vi "Add Shared Variables.vi"(8 "error in (no error)":errorcluster, 11 "Node Ptr":u64 format="%.0x") -> (0 "error out":errorcluster)   [LabVIEW 2017]
uses:
  Support/Add SV Process/Channel Configuration States.ctl
  Support/ChannelVS/ChannelVS.lvclass
  C:/Users/Public/Documents/National Instruments/NI VeriStand 2017/Custom Devices/Shared Variables CD 2.0/Data/Channel.lvlibp/Channel.lvclass
  <vilib>/Utility/VariantDataType/Type.ctl
  Support/ChannelVS/ChannelVS.lvclass/ChannelVS.ctl
  Support/ChannelVS/Compare Ch with Ch List.vi
  Support/ChannelVS/Read VeriSTAND Channel Info.vi
  Support/ChannelVS/Write VeriSTAND Channel Info.vi
  Shared/SV Global.vi
  Public/Documents/National Instruments/NI VeriStand 2017/Custom Devices/Shared Variables CD 2.0/Data/Channel.lvlibp/Read Channel Info.vi
  <vilib>/NI VeriStand/Custom Device API/Custom Device API.lvlib
  Shared Variables CD 2.0 Configuration.lvlib
  <vilib>/Utility/VariantDataType/VariantType.lvlib
panel:
  out "Scope":string
  out "State":T1
  in  "Refresh Target":bool
  in  "Done":bool
  in  "Help":bool
  in  "Remove Button":bool
  in  "Add Button":bool
  in  "Target IPAddr":string caption="Target IP Address*"
  in  "CD List":string[](tree)
  in  "Target List":string[](tree)
  in  "Tag":string
  # "Manage Shared Variables to"
  # "*Do Not Use \"localhost\" or host name"
  # "*Grayed out variables are already added to Veristand"
  # "All Numeric data types will be handled as\nDouble Floating Point in VeriSTAND"
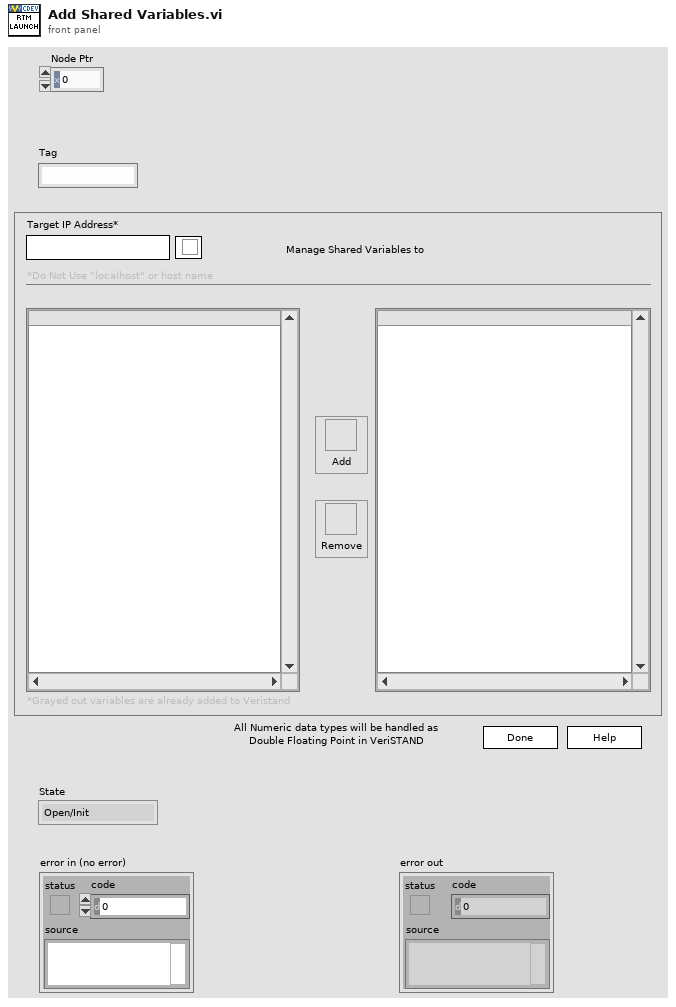
[diagram p1: front panel]
types:
  T1 = typedef "Shared Variables CD 2.0 Configuration.lvlib/Channel Configuration States.ctl" = enum16{"Open/Init", "Start Update", "Get VS Channels", "Get Available Ch from Target", "Wait On User Action", "Update Target Tree", "Update VS Trees", "Update Done", "Create VS Channels", "Remove VS Channels", "Error", "Close"}
  T2 = cluster{"Read Channel Array":refnum<class "ChannelVS.lvclass">[], "Write Channel Array":refnum<class "ChannelVS.lvclass">[]}
  T3 = typedef "Custom Device API.lvlib/Custom Device Item Info.ctl" = cluster{"Name":string, "Is Channel":bool, "GUID":string, "Is Waveform":bool}
  T4 = typedef "Custom Device API.lvlib/Custom Device Item Ref.ctl" = u64
  T5 = enum8{"Enabled", "Disabled", "Disabled and Grayed Out"}
  T6 = typedef "VariantType.lvlib/Type.ctl" = enum8{"Invalid Type", "Void", "I8", "I16", "I32", "I64", "U8", "U16", "U32", "U64", "Single Float", "Double Float", "Extended Float", "Single Complex", "Double Complex", "Extended Complex", "Enum U8", "Enum U16", "Enum U32", "Enum U64", "Single Float With Unit", "Double Float With Unit", "Extended Float With Unit", "Single Complex with Unit", "Double Complex with Unit", "Extended Complex with Unit", "Boolean", "String", "Path", "Picture", "Tag", "Array", "Cluster", "Variant", "LV Variant", "Waveform", "Timestamp", "Digital Waveform", "Digital Data", "ExpressData", "Refnum", "External Data", "VI", "Poly VI", "LabVIEW Class Instance", "Fixed Point"}
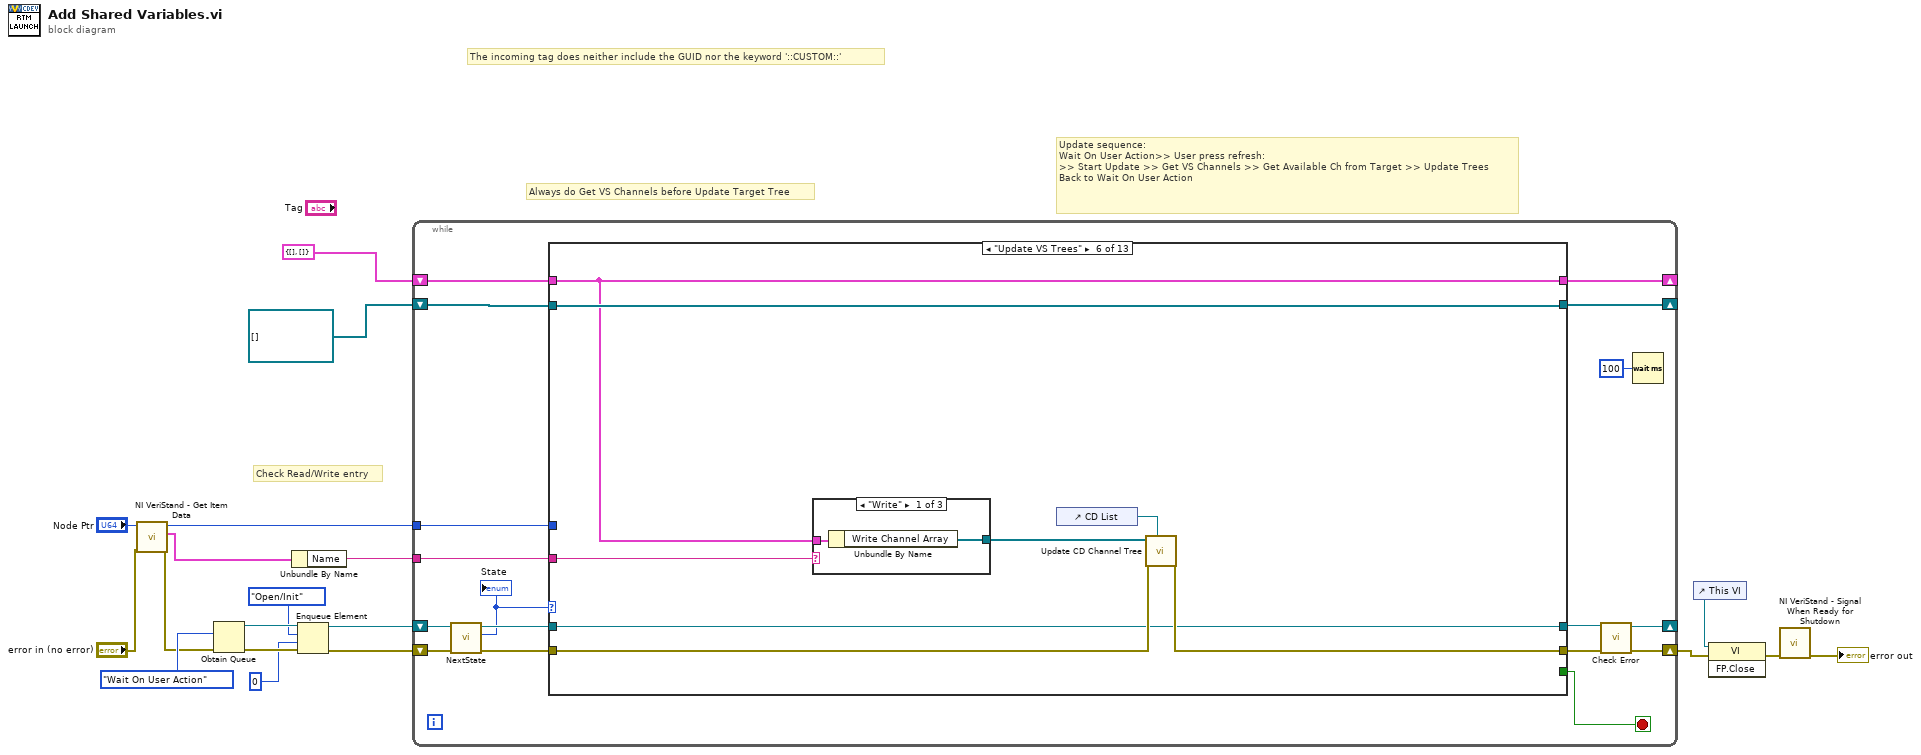
[diagram p0: block diagram]
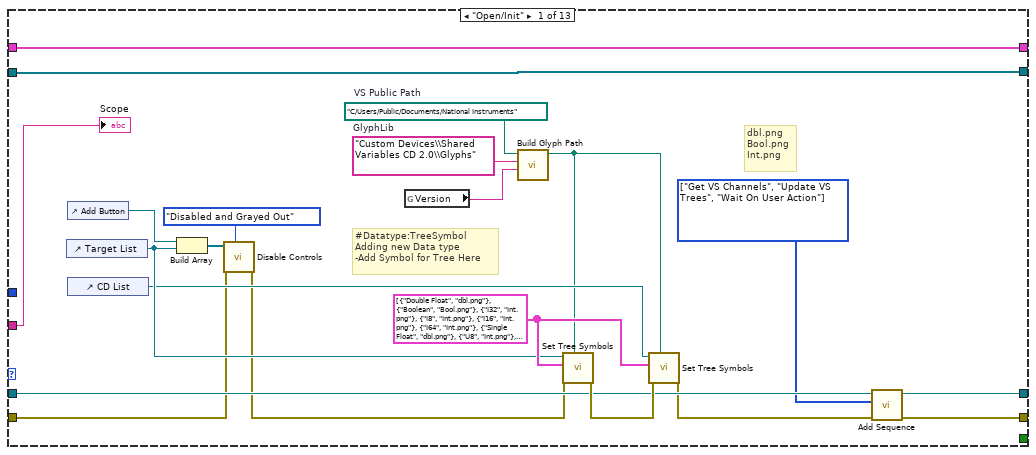
[diagram p2: hidden frame]
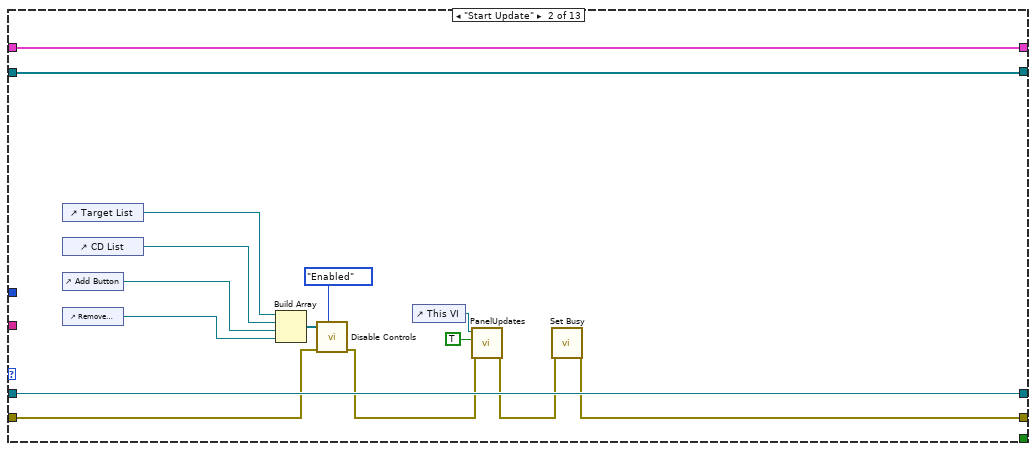
[diagram p3: hidden frame]
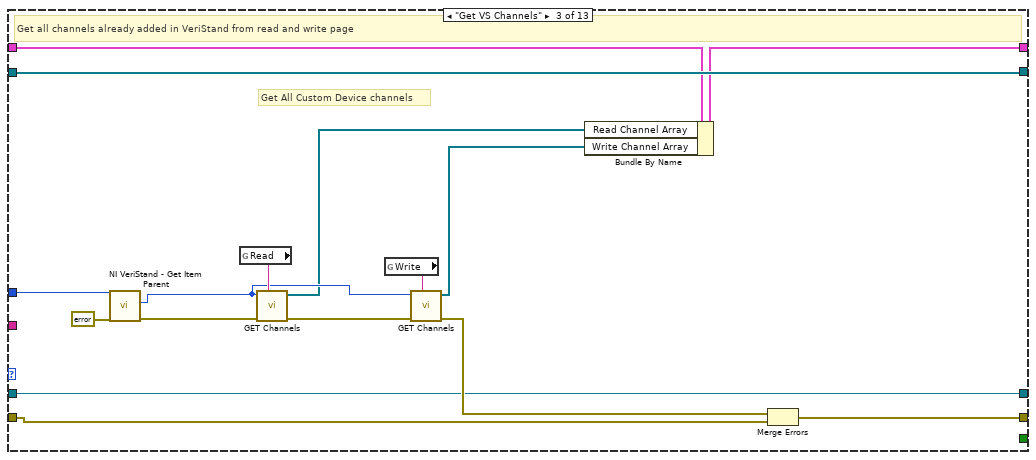
[diagram p4: hidden frame]
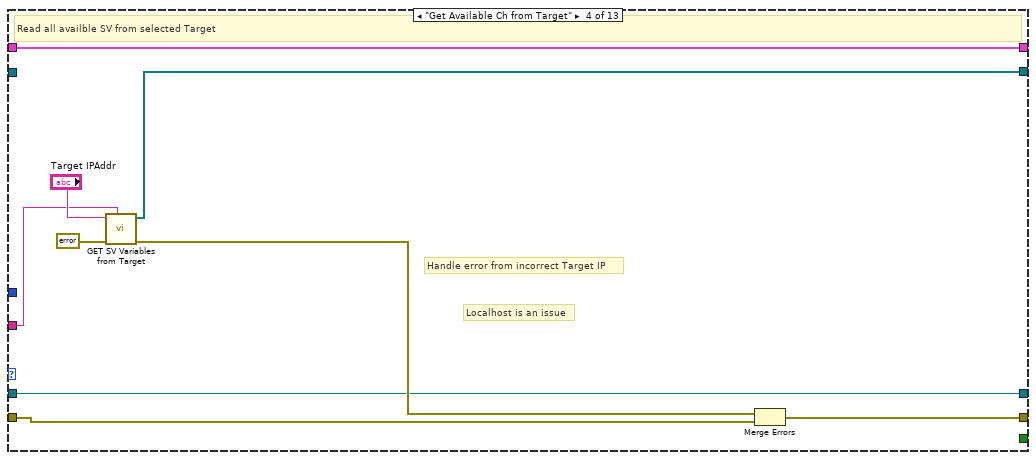
[diagram p5: hidden frame]
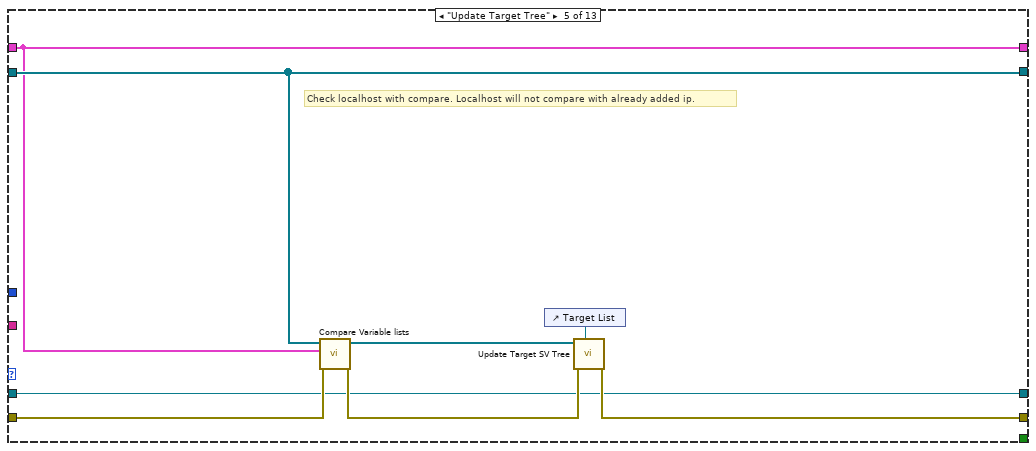
[diagram p6: hidden frame]
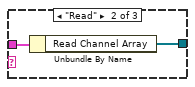
[diagram p7: hidden frame]
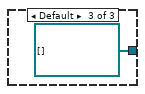
[diagram p8: hidden frame]
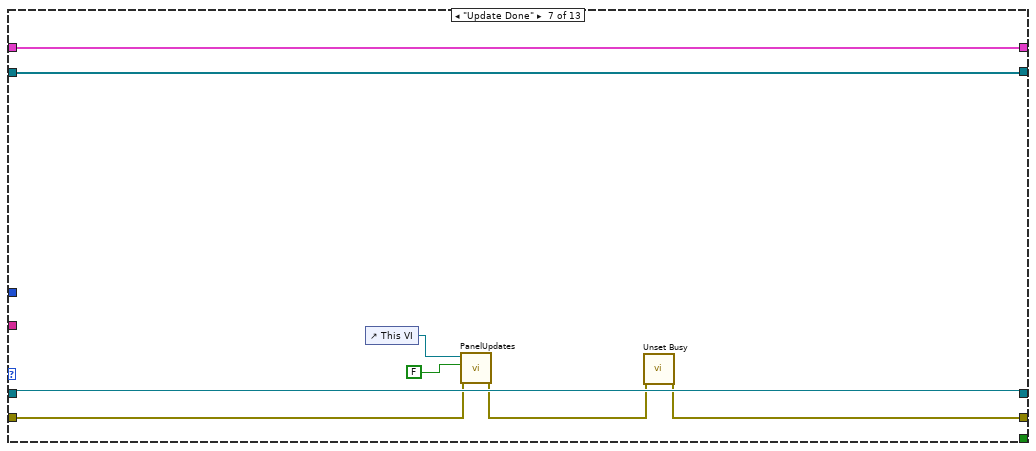
[diagram p9: hidden frame]
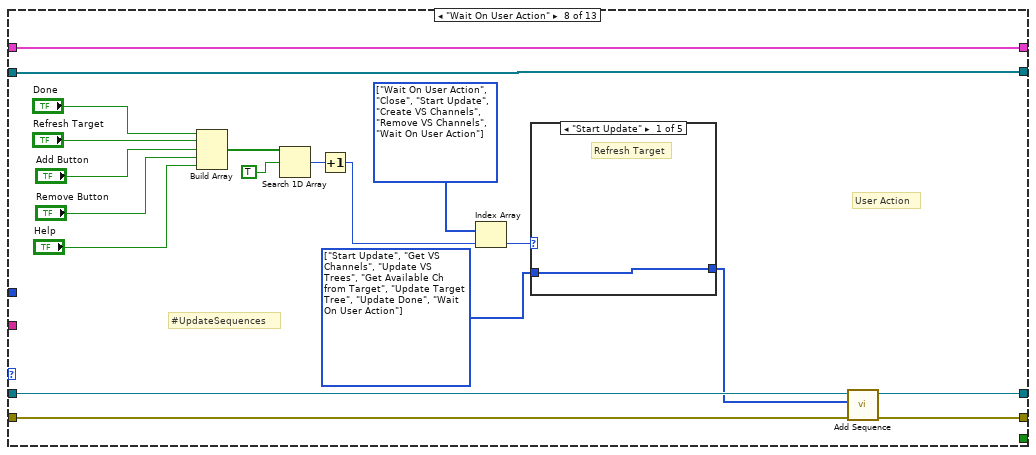
[diagram p10: hidden frame]
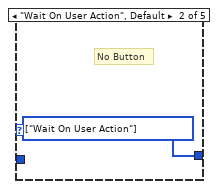
[diagram p11: hidden frame]
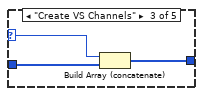
[diagram p12: hidden frame]
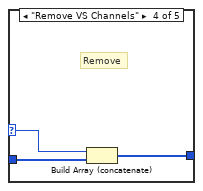
[diagram p13: hidden frame]
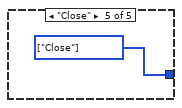
[diagram p14: hidden frame]
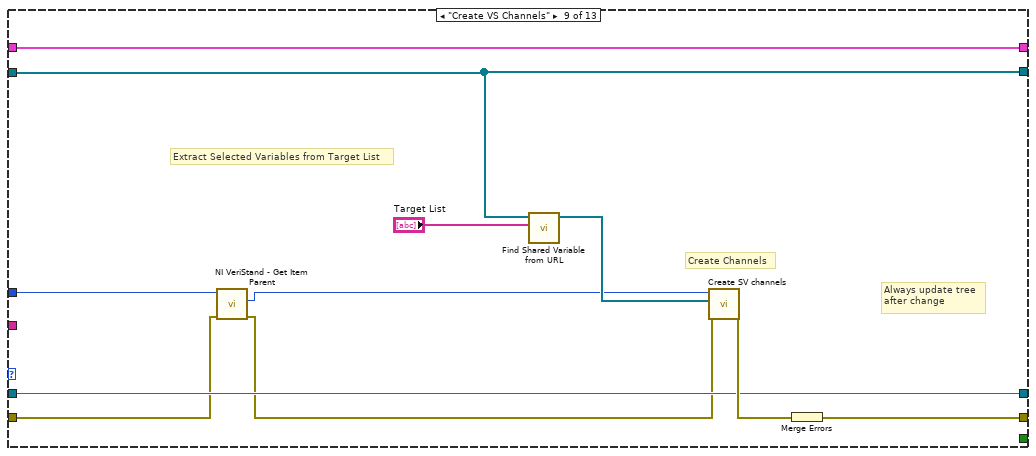
[diagram p15: hidden frame]
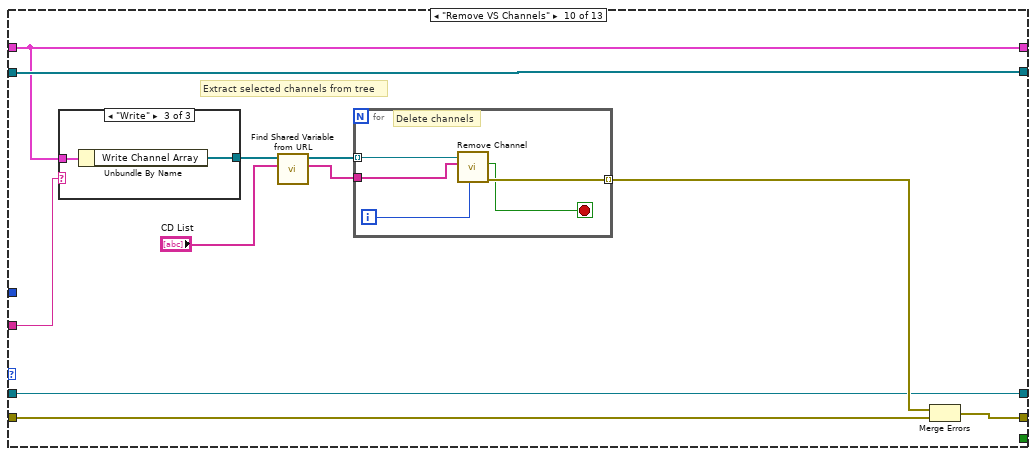
[diagram p16: hidden frame]
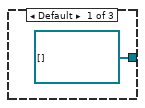
[diagram p17: hidden frame]
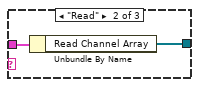
[diagram p18: hidden frame]
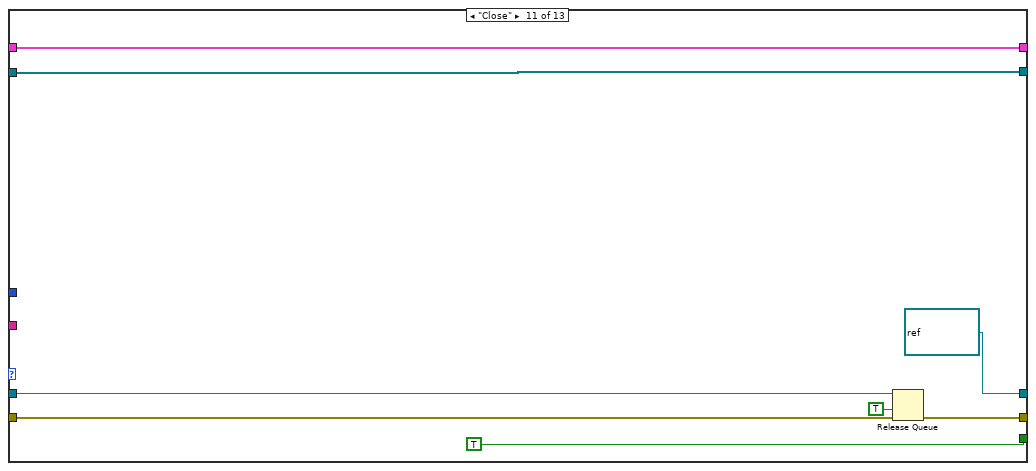
[diagram p19: hidden frame]
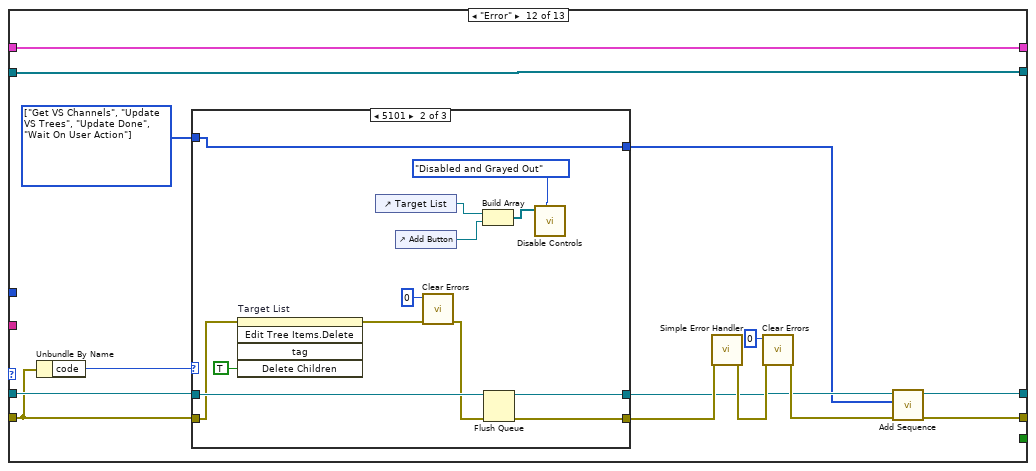
[diagram p20: hidden frame]
diagram:
  # "Always do Get VS Channels before Update Target Tree"
  # "Check Read/Write entry"
  # "Update sequence:\nWait On User Action>> User press refresh:\n>> Start Update >> Get VS Channels >> Get Available Ch from Target >> Update Trees\nBack to Wait On User Action"
  # "The incoming tag does neither include the GUID nor the keyword '::CUSTOM::'"
  n1 = call <vilib>:"NI VeriStand - Get Item Data.vi"("error in (no error)"="error in (no error)", "Item Ref in"="Node Ptr") -> ("error out"=w3:errorcluster, "Item Info"=w19:T3, "Item Ref out"=w16:T4)  [unwired: 6 in, 1 out]
  n2 = Obtain Queue(element data type=Channel_Configuration_States."Wait On User Action", error in (no error)=w3) -> (queue out=w7:refnum<queue>, error out=w6:errorcluster)  [unwired: 3 in, 1 out]
  n3 = Unbundle By Name(w19) -> ("Name"=w18:string)
  n4 = Enqueue Element(queue=w7, element=Channel_Configuration_States."Open/Init", timeout in ms (-1)=0, error in (no error)=w6) -> (queue out=w4:refnum<queue>, error out=w2:errorcluster)  [unwired: 1 out]
  n5 = while {
    tunnel: w18 -> [w20]
    tunnel: w16 -> [w36]
    shift-right: [w28] -> w17
    shift-left: w2 -> [w21]
    shift-right: [w35] -> _
    shift-left: T2 {"Read Channel Array"=[], "Write Channel Array"=[]} -> [w34]
    shift-right: [w32] -> _
    shift-left: refnum<class "ChannelVS.lvclass">[] [] ("Variable List") -> [w31]
    shift-right: [w23] -> _
    shift-left: w4 -> [w27]
    stop <- w33 stop-if-true
    n6 = call "NextState.vi"("error in (no error)"=w21, "Queue in"=w27) -> ("error out"=w22:errorcluster, "Next State"=w25:T1, "Queue out"=w26:refnum<queue>)  [unwired: 7 in]
    "State" <- w25
    n7 = case shown="\"Update VS Trees\"" w25 {
      tunnel: w22 -> [w43 w59 w82 w93 w103 w111 w123 w134 w158 w176 w191 w204 w241]
      tunnel: [w46 w60 w83 w94 w105 w110 w119 w133 w162 w173 w190 w198 w241] -> w29
      tunnel: w36 -> [_ _ w87 _ _ _ _ _ w164 _ _ _ _]
      tunnel: [w57 w72 w86 w97 w100 w112 w126 w145 w165 w174 w193 w208 w240] -> w35
      tunnel: w34 -> [w57 w72 w85 w97 w100 w112 w126 w145 w165 w174 w193 w208 w240]
      tunnel: [_ _ _ _ _ _ _ _ _ _ TRUE _ _] -> w33
      tunnel: [w56 w71 w88 w89 w101 w113 w125 w144 w155 w175 w192 w207 w239] -> w32
      tunnel: w31 -> [w56 w71 w88 _ w101 w113 w125 w144 w155 w175 w192 w207 w239]
      tunnel: w26 -> [w48 w64 w80 w92 w102 w109 w124 w132 w161 w171 w189 w205 w238]
      tunnel: [w47 w64 w80 w92 w102 w109 w124 w131 w161 w171 w187 w196 w238] -> w24
      tunnel: w20 -> [w37 _ _ w90 _ w108 _ _ _ w168 _ _ _]
      frame "Open/Init" {
        w40 = path "C:/Users/Public/Documents/National Instruments"  # VS Public Path
        w41 = "Custom Devices\\Shared Variables CD 2.0\\Glyphs"  # GlyphLib
        w44 = T1[] [enum."Get VS Channels", enum."Update VS Trees", enum."Wait On User Action"] items=["Open/Init", "Start Update", "Get VS Channels", "Get Available Ch from Target", "Wait On User Action", "Update Target Tree", "Update VS Trees", "Update Done", "Create VS Channels", "Remove VS Channels", "Error", "Close"]
        w53 = cluster{"Type":T6, string}[] [{"Type"=enum."Double Float", "dbl.png"}, {"Type"=enum."Boolean", "Bool.png"}, {"Type"=enum."I32", "Int.png"}, {"Type"=enum."I8", "Int.png"}, {"Type"=enum."I16", "Int.png"}, {"Type"=enum."I64", "Int.png"}, {"Type"=enum."Single Float", "dbl.png"}, {"Type"=enum."U8", "Int.png"}, {"Type"=enum."U16", "Int.png"}, {"Type"=enum."U32", "Int.png"}, {"Type"=enum."U64", "Int.png"}]
        # "dbl.png\nBool.png\nInt.png"
        # "#Datatype:TreeSymbol\nAdding new Data type\n-Add Symbol for Tree Here"
        n8 = control-ref of="Target List"() -> (w52:refnum<vi>)
        n9 = control-ref of="Add Button"() -> (w50:refnum<vi>)
        n10 = control-ref of="CD List"() -> (w49:refnum<vi>)
        n11 = Build Array(w50, w52) -> (w54:refnum<vi>[])
        n12 = call "Disable Controls.vi"("Disabled"=T5."Disabled and Grayed Out", "error in (no error)"=w43, "Array"=w54) -> ("error out"=w42:errorcluster)  [unwired: 8 in]
        n13 = global read "SV Global.vi" "Version"() -> (w38:string)
        n14 = call "Build Glyph Path.vi"("Version"=w38, "GlyphLib"=w41, "VS Public Path"=w40) -> ("Path to Glyph Lib"=w39:path)  [unwired: 8 in]
        n15 = call "Set Tree Symbols.vi"("Path to PNG lib"=w39, "error in (no error)"=w42, "Index and Image"=w53, "TreeControl in"=w52) -> ("error out"=w51:errorcluster)  [unwired: 7 in]
        n16 = call "Set Tree Symbols.vi"("Path to PNG lib"=w39, "error in (no error)"=w51, "Index and Image"=w53, "TreeControl in"=w49) -> ("error out"=w45:errorcluster)  [unwired: 7 in]
        n17 = call "Add Sequence.vi"("error in (no error)"=w45, "Transition Sequence"=w44, "Queue in"=w48) -> ("error out"=w46:errorcluster, "Queue out"=w47:refnum<queue>)  [unwired: 7 in]
        "Scope" <- w37
      }
      frame "Start Update" {
        n18 = control-ref of="Target List"() -> (w68:refnum<vi>)
        n19 = control-ref of="CD List"() -> (w69:refnum<vi>)
        n20 = control-ref of="Add Button"() -> (w70:refnum<vi>)
        n21 = control-ref of="Remove Button"() -> (w66:refnum<vi>)
        n22 = Build Array(w68, w69, w70, w66) -> (w65:refnum<vi>[])
        n23 = call "Disable Controls.vi"("Disabled"=T5."Enabled", "error in (no error)"=w59, "Array"=w65) -> ("error out"=w58:errorcluster)  [unwired: 8 in]
        n24 = control-ref of="This VI"() -> (w62:refnum<vi>)
        n25 = call "PanelUpdates.vi"("error in (no error)"=w58, "Defer Panel Updates"=TRUE, "VI in"=w62) -> ("error out"=w61:errorcluster)  [unwired: 8 in]
        n26 = call <vilib>:"Set Busy.vi"("error in (no error)"=w61) -> ("error out"=w60:errorcluster)  [unwired: 9 in, 1 out]
      }
      frame "Get VS Channels" {
        # "Get All Custom Device channels"
        # "Get all channels already added in VeriStand from read and write page"
        n27 = call <vilib>:"NI VeriStand - Get Item Parent.vi"("error in (no error)"=errorcluster {"status"=FALSE, "code"=0, "source"=""}, "Item Ref in"=w87) -> ("error out"=w77:errorcluster, "Parent Ref"=w75:T4)  [unwired: 6 in, 2 out]
        n28 = global read "SV Global.vi" "Read"() -> (w78:string)
        n29 = call "GET Channels.vi"("Channel Direction"=w78, "error in (no error)"=w77, "Item Ref in"=w75) -> ("error out"=w76:errorcluster, "VS Channel Array"=w74:refnum<class "ChannelVS.lvclass">[])  [unwired: 7 in]
        n30 = global read "SV Global.vi" "Write"() -> (w79:string)
        n31 = call "GET Channels.vi"("Channel Direction"=w79, "error in (no error)"=w76, "Item Ref in"=w75) -> ("error out"=w84:errorcluster, "VS Channel Array"=w73:refnum<class "ChannelVS.lvclass">[])  [unwired: 7 in]
        n32 = Bundle By Name(cluster=w85, "Read Channel Array"=w74, "Write Channel Array"=w73) -> (w86:T2)
        n33 = Merge Errors(w84, w82) -> (w83:errorcluster)
      }
      frame "Get Available Ch from Target" {
        # "Localhost is an issue"
        # "Handle error from incorrect Target IP"
        # "Read all availble SV from selected Target"
        n34 = call "GET SV Variables from Target.vi"("Read/Write"=w90, "error in (no error)"=errorcluster {"status"=FALSE, "code"=0, "source"=""}, "Target"="Target IPAddr") -> ("error out"=w96:errorcluster, "Channel Array"=w89:refnum<class "ChannelVS.lvclass">[])  [unwired: 7 in]
        n35 = Merge Errors(w96, w93) -> (w94:errorcluster)
      }
      frame "Update Target Tree" {
        # "Check localhost with compare. Localhost will not compare with already added ip."
        n36 = call "Compare Variable lists.vi"("error in (no error)"=w103, "Channel Arrays"=w100, "Variable List"=w101) -> ("error out"=w104:errorcluster, "Variable list compared"=w98:refnum<class "ChannelVS.lvclass">[])  [unwired: 7 in]
        n37 = control-ref of="Target List"() -> (w99:refnum<vi>)
        n38 = call "Update Target SV Tree.vi"("TreeControl in"=w99, "error in (no error)"=w104, "Variable list compared"=w98) -> ("error out"=w105:errorcluster)  [unwired: 8 in]
      }
      frame "Update VS Trees" {
        n39 = case shown="\"Write\"" w108 {
          tunnel: [w115 w116 refnum<class "ChannelVS.lvclass">[] [] ("Read Channel Array")] -> w107
          tunnel: w112 -> [w114 w117 _]
          frame "Write" {
            n40 = Unbundle By Name(w114) -> ("Write Channel Array"=w115:refnum<class "ChannelVS.lvclass">[])
          }
          frame "Read" {
            n41 = Unbundle By Name(w117) -> ("Read Channel Array"=w116:refnum<class "ChannelVS.lvclass">[])
          }
          frame Default {
          }
        }
        n42 = control-ref of="CD List"() -> (w106:refnum<vi>)
        n43 = call "Update CD Channel Tree.vi"("CD List"=w106, "error in (no error)"=w111, "Channel Array"=w107) -> ("error out"=w110:errorcluster)  [unwired: 8 in]
      }
      frame "Update Done" {
        n44 = control-ref of="This VI"() -> (w122:refnum<vi>)
        n45 = call "PanelUpdates.vi"("error in (no error)"=w123, "Defer Panel Updates"=FALSE, "VI in"=w122) -> ("error out"=w120:errorcluster)  [unwired: 8 in]
        n46 = call <vilib>:"Unset Busy.vi"("error in (no error)"=w120) -> ("error out"=w119:errorcluster)  [unwired: 10 in]
      }
      frame "Wait On User Action" {
        w127 = T1[] [enum."Wait On User Action", enum."Close", enum."Start Update", enum."Create VS Channels", enum."Remove VS Channels", enum."Wait On User Action"] items=["Open/Init", "Start Update", "Get VS Channels", "Get Available Ch from Target", "Wait On User Action", "Update Target Tree", "Update VS Trees", "Update Done", "Create VS Channels", "Remove VS Channels", "Error", "Close"]
        w128 = T1[] [enum."Start Update", enum."Get VS Channels", enum."Update VS Trees", enum."Get Available Ch from Target", enum."Update Target Tree", enum."Update Done", enum."Wait On User Action"] items=["Open/Init", "Start Update", "Get VS Channels", "Get Available Ch from Target", "Wait On User Action", "Update Target Tree", "Update VS Trees", "Update Done", "Create VS Channels", "Remove VS Channels", "Error", "Close"]
        # "#UpdateSequences"
        # "User Action"
        n47 = Build Array("Done", "Refresh Target", "Add Button", "Remove Button", "Help") -> (w138:bool[])
        n48 = Search 1D Array(1D array=w138, element=TRUE) -> (index of element=w136:i32)  [unwired: 1 in]
        n49 = Increment(x=w136) -> (x+1=w135:i32)
        n50 = Index Array(array=w127, index=w135) -> (element=w130:T1)
        n51 = case shown="\"Start Update\"" w130 {
          selector: w130 -> [_ _ w149 w152 _]
          tunnel: [w146 w147 w148 w151 w154] -> w129
          tunnel: w128 -> [w146 _ w150 w153 _]
          frame "Start Update" {
            # "Refresh Target"
          }
          frame "Wait On User Action", Default {
            w147 = T1[] [enum."Wait On User Action"] items=["Open/Init", "Start Update", "Get VS Channels", "Get Available Ch from Target", "Wait On User Action", "Update Target Tree", "Update VS Trees", "Update Done", "Create VS Channels", "Remove VS Channels", "Error", "Close"]
            # "No Button"
          }
          frame "Create VS Channels" {
            n52 = Build Array (concatenate)(w149, w150) -> (w148:T1[])
          }
          frame "Remove VS Channels" {
            # "Remove"
            n53 = Build Array (concatenate)(w152, w153) -> (w151:T1[])
          }
          frame "Close" {
            w154 = T1[] [enum."Close"] items=["Open/Init", "Start Update", "Get VS Channels", "Get Available Ch from Target", "Wait On User Action", "Update Target Tree", "Update VS Trees", "Update Done", "Create VS Channels", "Remove VS Channels", "Error", "Close"]
          }
        }
        n54 = call "Add Sequence.vi"("error in (no error)"=w134, "Transition Sequence"=w129, "Queue in"=w132) -> ("error out"=w133:errorcluster, "Queue out"=w131:refnum<queue>)  [unwired: 7 in]
      }
      frame "Create VS Channels" {
        # "Create Channels"
        # "Extract Selected Variables from Target List"
        # "Always update tree\nafter change"
        n55 = call <vilib>:"NI VeriStand - Get Item Parent.vi"("error in (no error)"=w158, "Item Ref in"=w164) -> ("error out"=w157:errorcluster, "Parent Ref"=w156:T4)  [unwired: 6 in, 2 out]
        n56 = call "Find Shared Variable from URL.vi"("Target List"="Target List", "Variable List"=w155) -> ("Variable info"=w159:refnum<class "ChannelVS.lvclass">[])  [unwired: 8 in, 1 out]
        n57 = call "Create SV channels.vi"("error in"=w157, "Variable List"=w159, "Custom Device in"=w156) -> ("error out"=w163:errorcluster)  [unwired: 7 in, 1 out]
        n58 = Merge Errors(w163) -> (w162:errorcluster)
      }
      frame "Remove VS Channels" {
        # "Extract selected channels from tree"
        n59 = case shown="\"Write\"" w168 {
          tunnel: w174 -> [_ w184 w186]
          tunnel: [refnum<class "ChannelVS.lvclass">[] [] ("Write Channel Array") w183 w185] -> w167
          frame Default {
          }
          frame "Read" {
            n60 = Unbundle By Name(w184) -> ("Read Channel Array"=w183:refnum<class "ChannelVS.lvclass">[])
          }
          frame "Write" {
            n61 = Unbundle By Name(w186) -> ("Write Channel Array"=w185:refnum<class "ChannelVS.lvclass">[])
          }
        }
        n62 = call "Find Shared Variable from URL.vi"("Target List"="CD List", "Variable List"=w167) -> ("Sort Name List"=w169:string[], "Variable info"=w166:refnum<class "ChannelVS.lvclass">[])  [unwired: 8 in]
        n63 = for {
          tunnel: [w181] -> w172 mode=indexing
          tunnel: w169 -> [w179]
          tunnel: w166 -> [w177] mode=indexing
          i -> [w180]
          stop <- w178 stop-if-true
          # "Delete channels"
          n64 = call "Remove Channel.vi"("Index from Loop Node (0)"=w180, "Name List"=w179, "ChannelVS in"=w177) -> ("error out"=w181:errorcluster, "Cancelled"=w178:bool)  [unwired: 7 in]
        }
        n65 = Merge Errors(w172, w176) -> (w173:errorcluster)
      }
      frame "Close" {
        w187 = refnum<queue> refnum items=["Open/Init", "Start Update", "Get VS Channels", "Get Available Ch from Target", "Wait On User Action", "Update Target Tree", "Update VS Trees", "Update Done", "Create VS Channels", "Remove VS Channels", "Error", "Close"] ("queue out")
        n66 = Release Queue(queue=w189, force destroy? (F)=TRUE, error in (no error)=w191) -> (error out=w190:errorcluster)  [unwired: 2 out]
      }
      frame "Error" {
        w202 = T1[] [enum."Get VS Channels", enum."Update VS Trees", enum."Update Done", enum."Wait On User Action"] items=["Open/Init", "Start Update", "Get VS Channels", "Get Available Ch from Target", "Wait On User Action", "Update Target Tree", "Update VS Trees", "Update Done", "Create VS Channels", "Remove VS Channels", "Error", "Close"]
        n67 = Unbundle By Name(w204) -> ("code"=w203:i32)
        n68 = case shown="5101" w203 {
          tunnel: [w214 w227 w237] -> w197
          tunnel: [w213 w226 w236] -> w201
          tunnel: w205 -> [w212 w225 w235]
          tunnel: w204 -> [w211 w224 w234]
          tunnel: [w209 w220 w233] -> w195
          tunnel: w202 -> [w209 w220 w233]
          frame 5100 {
            n69 = invoke on="Target List" class="Tree (strict)" method="Edit Tree Items.Delete"(error in=w211, "Delete Children"=TRUE ("Delete Children?")) -> (error out=w210:errorcluster)  [unwired: 3 in, 4 out]
            n70 = control-ref of="Target List"() -> (w217:refnum<vi>)
            n71 = control-ref of="Add Button"() -> (w216:refnum<vi>)
            n72 = Build Array(w217, w216) -> (w215:refnum<vi>[])
            n73 = Flush Queue(queue=w212, error in (no error)=w210) -> (queue out=w214:refnum<queue>, error out=w213:errorcluster)  [unwired: 1 out]
            n74 = call "Disable Controls.vi"("Disabled"=T5."Disabled and Grayed Out", "Array"=w215) -> ()  [unwired: 9 in, 1 out]
          }
          frame 5101 {
            n75 = invoke on="Target List" class="Tree (strict)" method="Edit Tree Items.Delete"(error in=w224, "Delete Children"=TRUE ("Delete Children?")) -> (error out=w223:errorcluster)  [unwired: 3 in, 4 out]
            n76 = control-ref of="Target List"() -> (w230:refnum<vi>)
            n77 = control-ref of="Add Button"() -> (w229:refnum<vi>)
            n78 = call <vilib>:"Clear Errors.vi"("error in (no error)"=w223, "specific error code to clear (0: all)"=0) -> ("error out"=w222:errorcluster)  [unwired: 4 in, 1 out]
            n79 = Build Array(w230, w229) -> (w228:refnum<vi>[])
            n80 = Flush Queue(queue=w225, error in (no error)=w222) -> (queue out=w227:refnum<queue>, error out=w226:errorcluster)  [unwired: 1 out]
            n81 = call "Disable Controls.vi"("Disabled"=T5."Disabled and Grayed Out", "Array"=w228) -> ()  [unwired: 9 in, 1 out]
          }
          frame Default {
            n82 = Flush Queue(queue=w235, error in (no error)=w234) -> (queue out=w237:refnum<queue>, error out=w236:errorcluster)  [unwired: 1 out]
          }
        }
        n83 = call <vilib>:"Simple Error Handler.vi"("error in (no error)"=w201) -> ("error out"=w206:errorcluster)  [unwired: 4 in, 4 out]
        n84 = call <vilib>:"Clear Errors.vi"("error in (no error)"=w206, "specific error code to clear (0: all)"=0) -> ("error out"=w199:errorcluster)  [unwired: 4 in, 1 out]
        n85 = call "Add Sequence.vi"("error in (no error)"=w199, "Transition Sequence"=w195, "Queue in"=w197) -> ("error out"=w198:errorcluster, "Queue out"=w196:refnum<queue>)  [unwired: 7 in]
      }
      frame Default {
      }
    }
    n86 = call "Check Error.vi"("error in (no error)"=w29, "queue in"=w24) -> ("error out"=w28:errorcluster, "queue out"=w23:refnum<queue>)  [unwired: 8 in]
    n87 = Wait (ms)(milliseconds to wait=u32 100) -> ()  [unwired: 1 out]
  }
  n88 = control-ref of="This VI"() -> (w11:refnum<vi>)
  n89 = invoke class="VI" method="FP.Close"(reference=w11, error in=w17) -> (error out=w13:errorcluster)  [unwired: 1 in, 2 out]
  n90 = call <vilib>:"NI VeriStand - Signal When Ready for Shutdown.vi"("error in (no error)"=w13) -> ("error out"=→"error out":errorcluster)  [unwired: 10 in]
